vi "2 Shift Goal.vi"   [LabVIEW 2011]
doc: "Multiplies drift velocity (from current and wind together) with estimated time that the boat will take to travel to the waypoint to determine how much to shift the goal location. The object is to shift the goal by the same amount as the total drift will be. The shift is applied to the waypoint location and each of it's no sail zones."
uses:
  2 Globals/2 Global.vi
  2 Classes/Waypoint/Waypoint.lvclass
  2 Typedefs/UTM Circle.ctl
types:
  T1 = typedef "UTM Circle.ctl" = cluster{"UTM Zone":dbl, "Hemisphere":enum16{"North", "South"}, "East":dbl, "North":dbl, "Radius":dbl}
  T2 = typedef "UTM Location.ctl" = cluster{"UTM Zone":dbl, "Hemisphere":enum16{"North", "South"}, "East":dbl, "North":dbl}
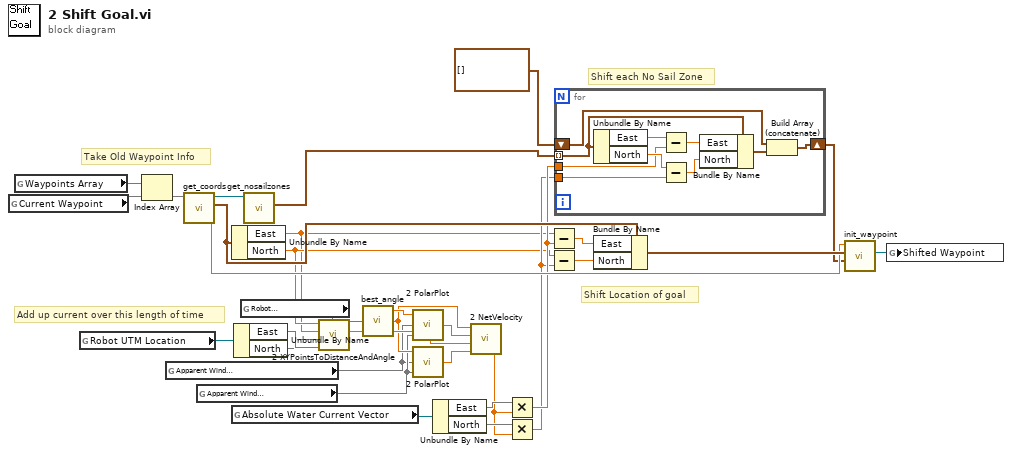
[diagram p0: block diagram]
diagram:
  # "Shift Location of goal"
  # "Add up current over this length of time"
  # "Take Old Waypoint Info"
  # "Shift each No Sail Zone"
  n1 = global read "2 Global.vi" "Current Waypoint"() -> (w32)
  n2 = global read "2 Global.vi" "Waypoints Array"() -> (w33)
  n3 = global read "2 Global.vi" "Robot UTM Location"() -> (w8:refnum<class "UTM_Location.lvclass">)
  n4 = Index Array(array=w33, index=w32) -> (element=w5)
  n5 = global read "2 Global.vi" "Apparent Wind\nDirection (º)"() -> (w1)
  n6 = call-dynamic "get_coords.vi"("Waypoint in"=w5) -> ("Tolerance (meters?)"=w16:dbl, "Coords"=w31:T2, "Waypoint out"=w18:refnum<class "Waypoint.lvclass">)  [unwired: 7 in, 1 out]
  n7 = global read "2 Global.vi" "Apparent Wind\nSpeed"() -> (w2)
  n8 = Unbundle By Name(w31) -> ("East"=w3:dbl, "North"=w4:dbl)
  n9 = global read "2 Global.vi" "Absolute Water Current Vector"() -> (w30:refnum<class "CartesianVector.lvclass">)
  n10 = Unbundle By Name(w8) -> ("East"=w7, "North"=w6)
  n11 = global read "2 Global.vi" "Robot\nHeading"() -> (w10)
  n12 = call-dynamic "get_nosailzones.vi"("Waypoint in"=w18) -> ("No Sail Circles"=w15:T1[])  [unwired: 7 in, 2 out]
  n13 = call "2 XYPointsToDistanceAndAngle.vi"("East 2"=w7, "North 2"=w6, "East 1"=w3, "North 1"=w4) -> ("Angle Diff"=w9:dbl)  [unwired: 6 in, 1 out]
  n14 = call "best_angle.vi"("Waypoint Heading"=w9, "Current Heading"=w10) -> ("Heading Candidate 2"=w24:dbl, "Heading Candidate 1"=w20:dbl, "Best Angle"=w21:dbl)  [unwired: 1 in]
  n15 = call "2 PolarPlot.vi"("Apparent Wind\nSpeed"=w2, "Apparent Wind\nDirection (º)"=w1, "Boat Angle"=w21) -> ("Velocity"=w23:dbl)
  n16 = call "2 PolarPlot.vi"("Apparent Wind\nSpeed"=w2, "Apparent Wind\nDirection (º)"=w1, "Boat Angle"=w20) -> ("Velocity"=w22:dbl)
  n17 = Unbundle By Name(w30) -> ("East"=w27, "North"=w26)
  n18 = call "2 NetVelocity.vi"("Speed 2"=w22, "Angle 2"=w24, "Speed 1"=w23, "Angle 1"=w20) -> ("Net Velocity"=w25:dbl)  [unwired: 7 in]
  n19 = Multiply(x=w27, y=w25) -> (x*y=w14:dbl)
  n20 = Multiply(x=w26, y=w25) -> (x*y=w13:dbl)
  n21 = Subtract(x=w3, y=w14) -> (x-y=w29:dbl)
  n22 = Subtract(x=w4, y=w13) -> (x-y=w28:dbl)
  n23 = for {
    tunnel: w15 -> [w42] mode=indexing
    tunnel: w14 -> [w35]
    tunnel: w13 -> [w34]
    shift-right: [w40] -> w11
    shift-left: T1[] [] -> [w43]
    n24 = Unbundle By Name(w42) -> ("East"=w37:dbl, "North"=w36:dbl)
    n25 = Subtract(x=w37, y=w35) -> (x-y=w38:dbl)
    n26 = Subtract(x=w36, y=w34) -> (x-y=w39:dbl)
    n27 = Bundle By Name(cluster=w42, "East"=w38, "North"=w39) -> (w41:T1)
    n28 = Build Array (concatenate)(w43, w41) -> (w40:T1[])
  }
  n29 = Bundle By Name(cluster=w31, "East"=w29, "North"=w28) -> (w19:T2)
  n30 = call "init_waypoint.vi"("No Sail Circles"=w11, "Coords"=w19, "Tolerance (m)"=w16) -> ("Waypoint Out"=w17:refnum<class "Waypoint.lvclass">)  [unwired: 8 in]
  n31 = global write "2 Global.vi" "Shifted Waypoint"(w17) -> ()
